vi "Julian_project7.vi"() -> ()   [LabVIEW 2020]
uses:
  <vilib>/imath/engines/lvmath2/RunTimeEngine/Managers/WorkSpace/UID Generator.vi
  <vilib>/imath/engines/lvmath2/RunTimeEngine/RunTimeType/NIMS_RunTimeType_From StrictType (excl LVString).vi
  <instcachedir>/0/NIMS_RunTimeType_From StrictType (excl LVString)_283B1B2000484AAA8744D21CE97EA49F.lvgen/NIMS_RunTimeType_From StrictType (excl LVString)_283B1B2000484AAA8744D21CE97EA49F_000.vi
  <vilib>/imath/engines/lvmath2/RunTimeEngine/LocalVariableDefStatement/MC_LocalVariableDefStatement_Display.vi
  <vilib>/imath/engines/lvmath2/RunTimeEngine/RangeToken/NIMS_Range.vi
  <instcachedir>/0/NIMS_Range_913EBD8295F041DB898D90A83F67761F.lvgen/NIMS_Range_913EBD8295F041DB898D90A83F67761F_000.vi
  <vilib>/imathl/engines/lvmath/Functions/Error Handling/Create Error.vi
  <vilib>/imath/engines/lvmath2/RunTimeEngine/Managers/SymbolTable/Clear UID.vi
  <vilib>/imath/engines/lvmath2/RunTimeEngine/NodeEndStatement/NIMS_NodeEndStatement_Output.vi
  <instcachedir>/0/NIMS_NodeEndStatement_Output_53EC0D466D134D7ABD903AC30B43404B.lvgen/NIMS_NodeEndStatement_Output_53EC0D466D134D7ABD903AC30B43404B_001.vi
  <instcachedir>/0/NIMS_NodeEndStatement_Output_53EC0D466D134D7ABD903AC30B43404B.lvgen/NIMS_NodeEndStatement_Output_53EC0D466D134D7ABD903AC30B43404B_005.vi
  <vilib>/imath/engines/lvmath2/RunTimeEngine/ErrorHandling/NIMS_Finalize Error.vi
  <vilib>/imath/engines/lvmath2/RunTimeEngine/Managers/SymbolTable/NIMS_WorkSpace.lvlib
  <vilib>/Analysis/NI_AAL_SigProc.lvlib
  <vilib>/Analysis/NI_AALPro.lvlib
panel:
  out "Distance In":dbl
  out "?":string
  out "?":string
  out "?":string
  out "Approximate \npower Curve 4":dbl[](graph) caption="Signals"
  out "Approximate power curve of V(t)":cluster{i32, i32, "Best Exponential Fit":dbl[]}(graph)
  out "Approximate power curve of A(t)":cluster{i32, dbl, "Best Exponential Fit":dbl[]}(graph)
  out "A(t) 2":cluster{"t_min":i32, "Ts":dbl, "y":dbl[]}(graph)
  out "Loop Iteration":i32
  out "Last 10k samples":dynamicdata(graph) caption="Signals"
  in  "?":bool
  in  "Given data or sampled data":bool
  in  "LPF cutoff":dbl=100.0 caption="Lower Cut-Off"
  in  "Sample Rate":dbl=1000.0 format="%#_13g"
  out "Calculated DC offset":dbl format="%#_13g"
  in  "Mode":bool
  out "X(t)":cluster{"t_min":i32, "Ts":dbl, "y":dbl[]}(graph)
  out "V(t)":cluster{"t_min":i32, "Ts":dbl, "y":dbl[]}(graph)
  # "Tyler Julian\nProject 7"
  # "Debug and Control"
  # "Sampled \nby Tyler"
  # "Example Data"
  # "Measurement"
  # "Simulation"
  # "Distance traveled."
  # "Acceleration"
  # "Velocity"
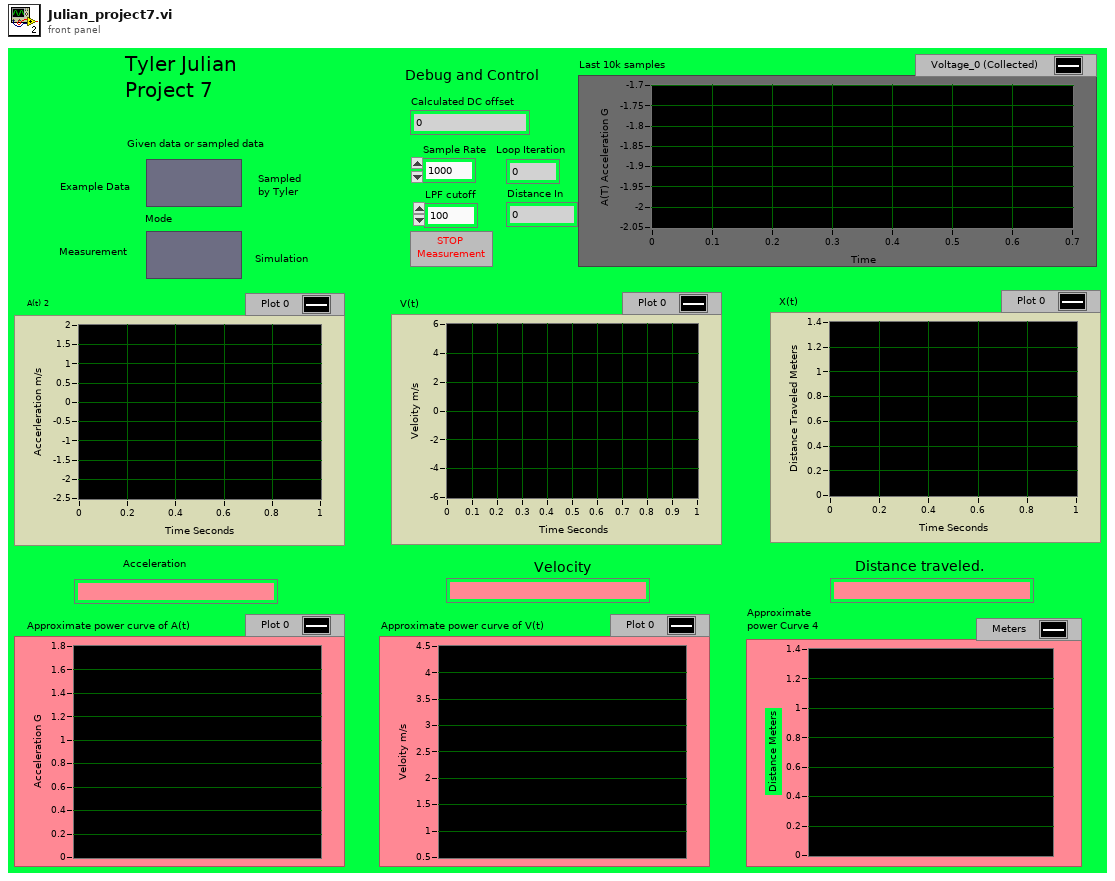
[diagram p1: front panel]
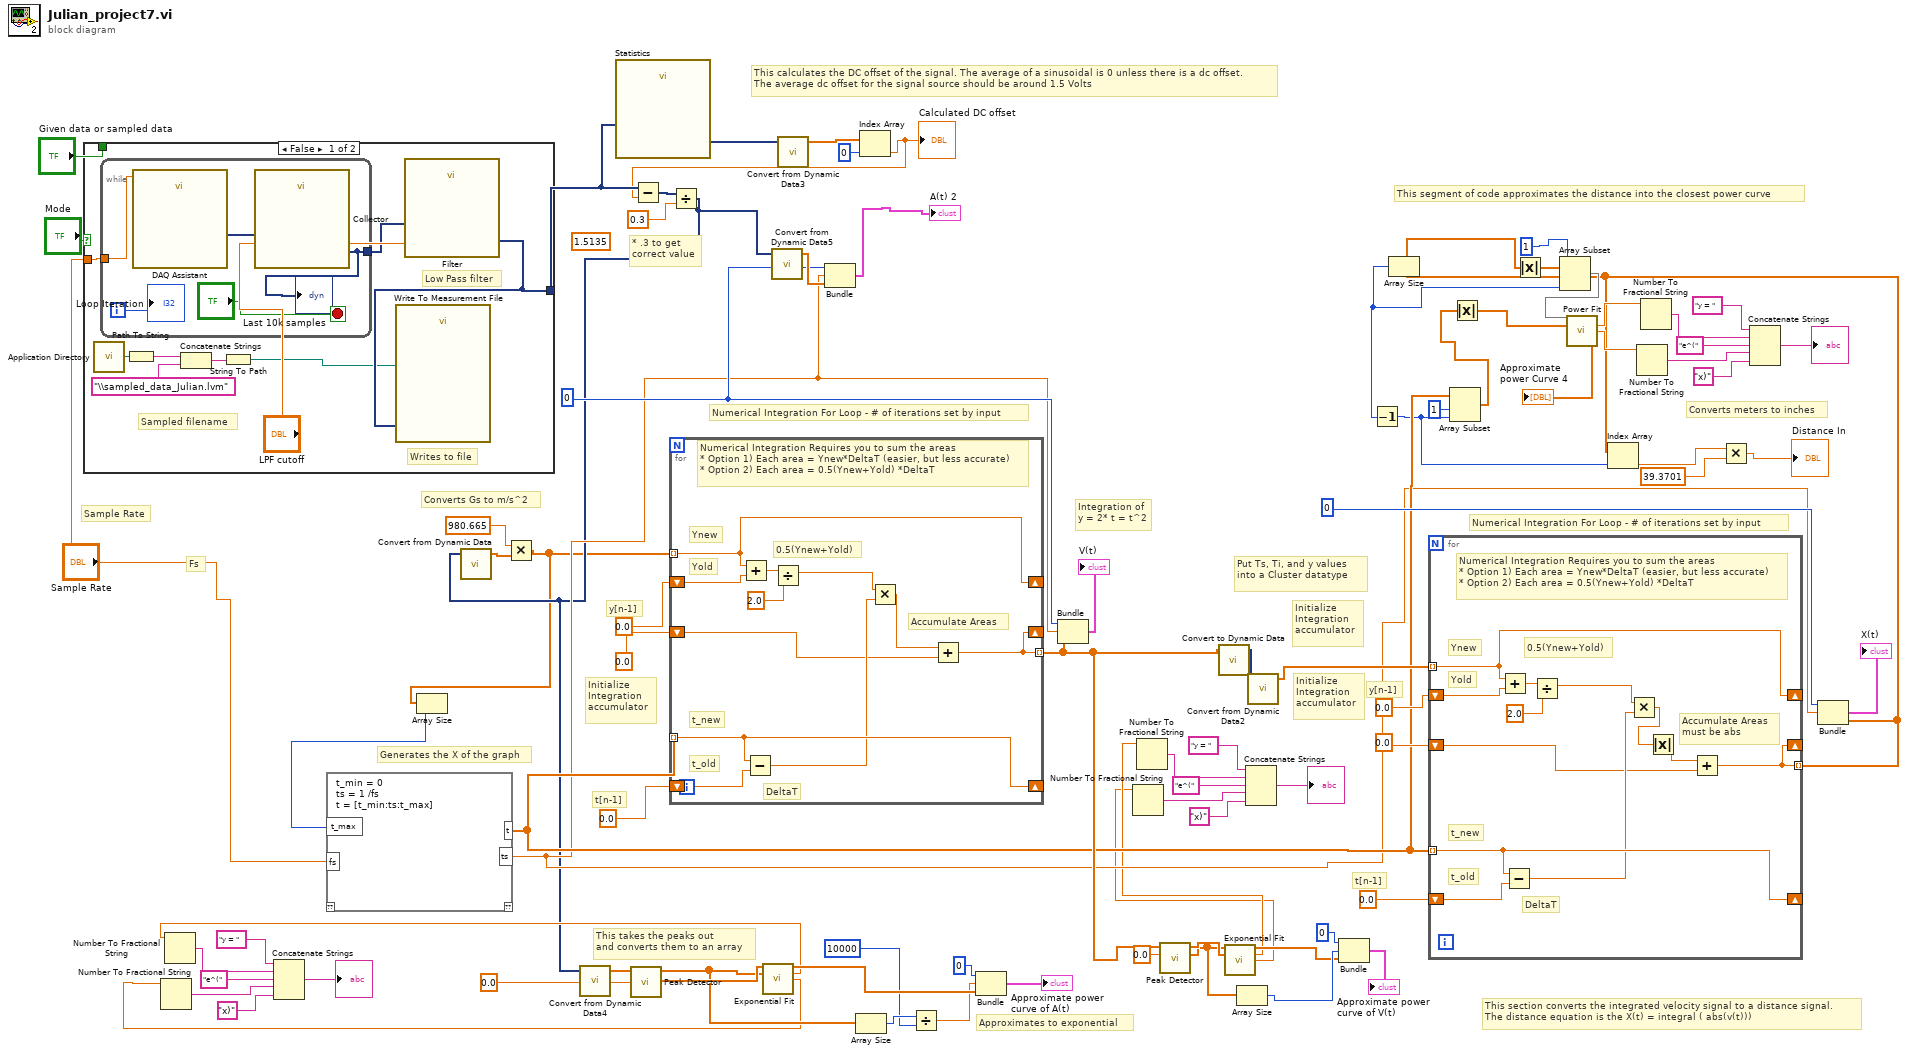
[diagram p0: block diagram]
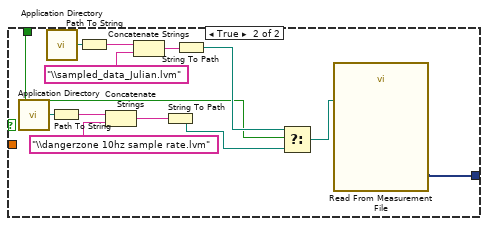
[diagram p2: hidden frame]
diagram:
  (unwired) 1.5135 ("y")
  w57 = 0
  # "Converts meters to inches"
  # "Converts Gs to m/s^2"
  # "Initialize\nIntegration\naccumulator"
  # "Initialize\nIntegration\naccumulator"
  # "Approximates to exponential"
  # "This segment of code approximates the distance into the closest power curve"
  # "* .3 to get \ncorrect value"
  # "This takes the peaks out \nand converts them to an array"
  # "Generates the X of the graph"
  # "Sample Rate"
  # "This calculates the DC offset of the signal. The average of a sinusoidal is 0 unless there is a dc offset.\nThe average dc offset for the signal source should be around 1.5 Volts"
  # "This section converts the integrated velocity signal to a distance signal. \nThe distance equation is the X(t) = integral ( abs(v(t)))"
  # "Put Ts, Ti, and y values into a Cluster datatype"
  # "Numerical Integration For Loop - # of iterations set by input"
  # "t[n-1]"
  # "y[n-1]"
  # "Fs"
  # "Integration of\ny = 2* t = t^2"
  # "Numerical Integration For Loop - # of iterations set by input"
  # "t[n-1]"
  # "y[n-1]"
  # "Initialize\nIntegration\naccumulator"
  n1 = case shown="False" "Mode" {
    tunnel: [w88 w109] -> w73
    tunnel: "Sample Rate" -> [w95 _]
    tunnel: "Given data or sampled data" -> [_ w102]
    frame False {
      # "Sampled filename"
      # "Writes to file"
      # "Low Pass filter"
      n2 = call <vilib>:"Application Directory.vi"() -> ("Application Directory"=w92:path)
      n3 = while {
        tunnel: w95 -> [w99]
        tunnel: [w97] -> w93
        i -> [w96]
        stop <- "?" stop-if-true
        n4 = call "DAQ Assistant"("rate"=w99) -> ("data"=w100:dynamicdata)  [unwired: 15 in, 3 out]
        n5 = call "Collector"("Signals"=w100) -> ("Collected Signals"=w97:dynamicdata)  [unwired: 9 in, 1 out]
        "Last 10k samples" <- w97
        "Loop Iteration" <- w96
      }
      n6 = Path To String(path=w92) -> (string=w91:string)
      n7 = Concatenate Strings(w91, "\\sampled_data_Julian.lvm" ("string")) -> (w89:string)
      n8 = String To Path(string=w89) -> (path=w87:path)
      n9 = call "Filter"("Lower Cut-Off"="LPF cutoff", "Signal"=w93) -> ("Filtered Signal"=w88:dynamicdata)  [unwired: 8 in, 1 out]
      n10 = call "Write To Measurement File"("Signals"=w88, "Filename"=w87) -> ()  [unwired: 15 in, 3 out]
    }
    frame True {
      n11 = call <vilib>:"Application Directory.vi"() -> ("Application Directory"=w113:path)
      n12 = call <vilib>:"Application Directory.vi"() -> ("Application Directory"=w106:path)
      n13 = Path To String(path=w113) -> (string=w112:string)
      n14 = Path To String(path=w106) -> (string=w107:string)
      n15 = Concatenate Strings(w112, "\\dangerzone 10hz sample rate.lvm" ("string")) -> (w110:string)
      n16 = Concatenate Strings(w107, "\\sampled_data_Julian.lvm" ("string")) -> (w108:string)
      n17 = String To Path(string=w110) -> (path=w103:path)
      n18 = String To Path(string=w108) -> (path=w104:path)
      n19 = Select(t=w104, s=w102, f=w103) -> (s? t:f=w101:path)
      n20 = call "Read From Measurement File"("Filename"=w101) -> ("Signals"=w109:dynamicdata)  [unwired: 5 in, 5 out]
    }
  }
  n21 = call "Statistics"("Signals"=w73) -> ("Arithmetic Mean"=w72:dynamicdata)  [unwired: 25 in, 1 out]
  n22 = call "Convert from Dynamic Data3"("Dynamic Data Type"=w72) -> ("Array"=w71:dbl[])  [unwired: 3 in]
  n23 = Index Array(array=w71, index=0) -> (element=w69:dbl)
  "Calculated DC offset" <- w69
  n24 = Subtract(x=w73, y=w69) -> (x-y=w85:dynamicdata)
  n25 = Divide(x=w85, y=0.3) -> (x/y=w9:dynamicdata)
  n26 = call "Convert from Dynamic Data"("Dynamic Data Type"=w9) -> ("Array"=w8:dbl[])  [unwired: 3 in]
  n27 = Multiply(x=980.665 ("t_min"), y=w8) -> (x*y=w7:dbl[])
  n28 = Array Size(array=w7) -> (size(s)=w66:i32)
  n29 = mathscript code="t_min = 0\nts = 1 /fs\nt = [t_min:ts:t_max]"("t_max"=w66, "fs"="Sample Rate") -> ("t"=w35:dbl[], "ts"=w34:dbl)  [unwired: 1 in, 1 out]
  n30 = call "Convert from Dynamic Data4"("Dynamic Data Type"=w9) -> ("Array"=w65:dbl[])  [unwired: 3 in]
  n31 = call <vilib>:"Peak Detector.vi"("threshold"=0.0, "X"=w65) -> ("Amplitudes"=w53:dbl[], "Locations"=w52:dbl[])  [unwired: 5 in, 3 out]
  n32 = for {
    shift-right: [w118] -> _
    shift-left: 0.0 ("t_min") -> [w119]
    tunnel: w7 -> [w117] mode=indexing
    shift-right: [w117] -> _
    shift-left: 0.0 ("t_min") -> [w124]
    tunnel: w35 -> [w122] mode=indexing
    shift-right: [w122] -> _
    shift-left: 0.0 ("t_min") -> [w123]
    tunnel: [w118] -> w63 mode=indexing
    # "0.5(Ynew+Yold)"
    # "Accumulate Areas"
    # "t_old"
    # "t_new"
    # "Yold"
    # "Ynew"
    # "DeltaT"
    # "Numerical Integration Requires you to sum the areas\n* Option 1) Each area = Ynew*DeltaT (easier, but less accurate)\n* Option 2) Each area = 0.5(Ynew+Yold) *DeltaT"
    n33 = Add(x=w117, y=w124) -> (x+y=w116:dbl)
    n34 = Subtract(x=w122, y=w123) -> (x-y=w121:dbl)
    n35 = Divide(x=w116, y=2.0) -> (x/y=w115:dbl)
    n36 = Multiply(x=w115, y=w121) -> (x*y=w120:dbl)
    n37 = Add(x=w120, y=w119) -> (x+y=w118:dbl)
  }
  n38 = call <vilib>:"Exponential Fit.vi"("Y"=w53, "X"=w52) -> ("Best Exponential Fit"=w56:dbl[], "amplitude"=w19:dbl, "damping"=w18:dbl)  [unwired: 8 in, 3 out]
  n39 = Number To Fractional String(number=w18) -> (F-format string=w22:string)  [unwired: 3 in]
  n40 = Number To Fractional String(number=w19) -> (F-format string=w24:string)  [unwired: 3 in]
  n41 = Concatenate Strings("y = " ("string"), w24, "e^(" ("string"), w22, "x)" ("string")) -> (→"?":string)
  n42 = call "Convert from Dynamic Data5"("Dynamic Data Type"=w9) -> ("Array"=w58:dbl[])  [unwired: 3 in]
  n43 = Bundle(w57, "ts"=w34, "Array"=w58) -> (→"A(t) 2":cluster{i32, "ts":dbl, "Array":dbl[]})  [unwired: 1 in]
  n44 = Array Size(array=w52) -> (size(s)=w51:i32)
  n45 = Divide(x=w51, y=10000) -> (x/y=w50:dbl)
  n46 = Bundle(0, w50, "Best Exponential Fit"=w56) -> (→"Approximate power curve of A(t)":cluster{i32, dbl, "Best Exponential Fit":dbl[]})  [unwired: 1 in]
  n47 = Bundle(w57, "ts"=w34, w63) -> (→"V(t)":cluster{i32, "ts":dbl, dbl[]})  [unwired: 1 in]
  n48 = call <vilib>:"Peak Detector.vi"("threshold"=0.0, "X"=w63) -> ("Amplitudes"=w46:dbl[], "Locations"=w61:dbl[])  [unwired: 5 in, 3 out]
  n49 = call "Convert to Dynamic Data"("Array"=w63) -> ("Dynamic Data Type"=w75:dynamicdata)  [unwired: 3 in]
  n50 = call <vilib>:"Exponential Fit.vi"("Y"=w46, "X"=w61) -> ("Best Exponential Fit"=w44:dbl[], "amplitude"=w11:dbl, "damping"=w10:dbl)  [unwired: 8 in, 3 out]
  n51 = Number To Fractional String(number=w10) -> (F-format string=w14:string)  [unwired: 3 in]
  n52 = Number To Fractional String(number=w11) -> (F-format string=w16:string)  [unwired: 3 in]
  n53 = Array Size(array=w46) -> (size(s)=w45:i32)
  n54 = Concatenate Strings("y = " ("string"), w16, "e^(" ("string"), w14, "x)" ("string")) -> (→"?":string)
  n55 = call "Convert from Dynamic Data2"("Dynamic Data Type"=w75) -> ("Array"=w77:dbl[])  [unwired: 3 in]
  n56 = Bundle(0, w45, "Best Exponential Fit"=w44) -> (→"Approximate power curve of V(t)":cluster{i32, i32, "Best Exponential Fit":dbl[]})  [unwired: 1 in]
  n57 = for {
    shift-right: [w131] -> _
    shift-left: 0.0 ("t_min") -> [w132]
    tunnel: w77 -> [w130] mode=indexing
    shift-right: [w130] -> _
    shift-left: 0.0 ("t_min") -> [w136]
    tunnel: w35 -> [w134] mode=indexing
    shift-right: [w134] -> _
    shift-left: 0.0 ("t_min") -> [w135]
    tunnel: [w131] -> w4 mode=indexing
    # "0.5(Ynew+Yold)"
    # "Accumulate Areas\nmust be abs"
    # "t_old"
    # "t_new"
    # "Yold"
    # "Ynew"
    # "DeltaT"
    # "Numerical Integration Requires you to sum the areas\n* Option 1) Each area = Ynew*DeltaT (easier, but less accurate)\n* Option 2) Each area = 0.5(Ynew+Yold) *DeltaT"
    n58 = Add(x=w130, y=w136) -> (x+y=w129:dbl)
    n59 = Subtract(x=w134, y=w135) -> (x-y=w133:dbl)
    n60 = Divide(x=w129, y=2.0) -> (x/y=w128:dbl)
    n61 = Multiply(x=w128, y=w133) -> (x*y=w126:dbl)
    n62 = Absolute Value(x=w126) -> (abs(x)=w125:dbl)
    n63 = Add(x=w125, y=w132) -> (x+y=w131:dbl)
  }
  n64 = Array Size(array=w4) -> (size(s)=w36:i32)
  n65 = Decrement(x=w36) -> (x-1=w5:i32)
  n66 = Array Subset(array=w35, index=1, length=w5) -> (w40:dbl[])
  n67 = Absolute Value(x=w40) -> (abs(x)=w41:dbl[])
  n68 = Absolute Value(x=w4) -> (abs(x)=w39:dbl[])
  n69 = Array Subset(array=w39, index=1, length=w36) -> (w37:dbl[])
  n70 = call <vilib>:"Power Fit.vi"("Y"=w37, "X"=w41) -> ("Best Power Fit"=→"Approximate \npower Curve 4":dbl[], "amplitude"=w33:dbl, "power"=w29:dbl)  [unwired: 8 in, 3 out]
  n71 = Index Array(array=w4, index=w5) -> (element=w3:dbl)
  n72 = Number To Fractional String(number=w29) -> (F-format string=w28:string)  [unwired: 3 in]
  n73 = Number To Fractional String(number=w33) -> (F-format string=w31:string)  [unwired: 3 in]
  n74 = Multiply(x=w3, y=39.3701) -> (x*y=→"Distance In":dbl)
  n75 = Concatenate Strings("y = " ("string"), w31, "e^(" ("string"), w28, "x)" ("string")) -> (→"?":string)
  n76 = Bundle(0, "ts"=w34, w4) -> (→"X(t)":cluster{i32, "ts":dbl, dbl[]})  [unwired: 1 in]
